vi "AlliGator Save Simulation Outputs to ASCII.vi"(8 "Error In":errorcluster, 11 "Fit Results":T1[](array[typedef])) -> (0 "Error Out":errorcluster)   [LabVIEW 2021, in "AlliGator Fit Method Benchmark.lvlib"]
doc: "Saves simulation results."
uses:
  AlliGator Fit Method Benchmark.lvlib
  Fits/IRF(X)PSED/IRF(X)PSED Fit Results.ctl
  Fits/IRF(X)PSED/Decay Fit Parameters & Derived Quantities List.ctl
  <vilib>/Utility/file.llb/Write Delimited Spreadsheet (DBL).vi
  Fits/Fits.lvlib
panel:
  out "Message":string
  # "see the AlliGator License on the block diagram (Ctrl+E or Window:Show Block Diagram)"
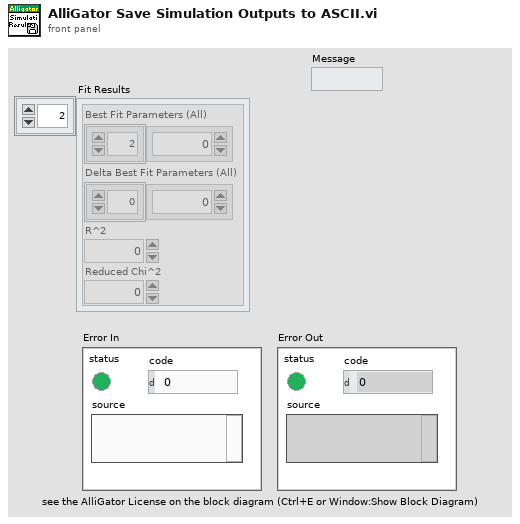
[diagram p1: front panel]
types:
  T1 = typedef "Fits.lvlib/IRF(X)PSED Fit Results.ctl" = cluster{"Best Fit Parameters (All)":dbl[], "Delta Best Fit Parameters (All)":dbl[], "R^2":dbl, "Reduced Chi^2":dbl}
  T2 = typedef "Fits.lvlib/Decay Fit Parameters & Derived Quantities List.ctl" = enum16{"Offset", "Baseline", "A_1", "tau_1", "A_2", "tau_2", "<tau>_a", "f1_a", "f2_a", "<tau>_i", "f1_i", "f2_i", "-", "R^2", "Chi^2"}
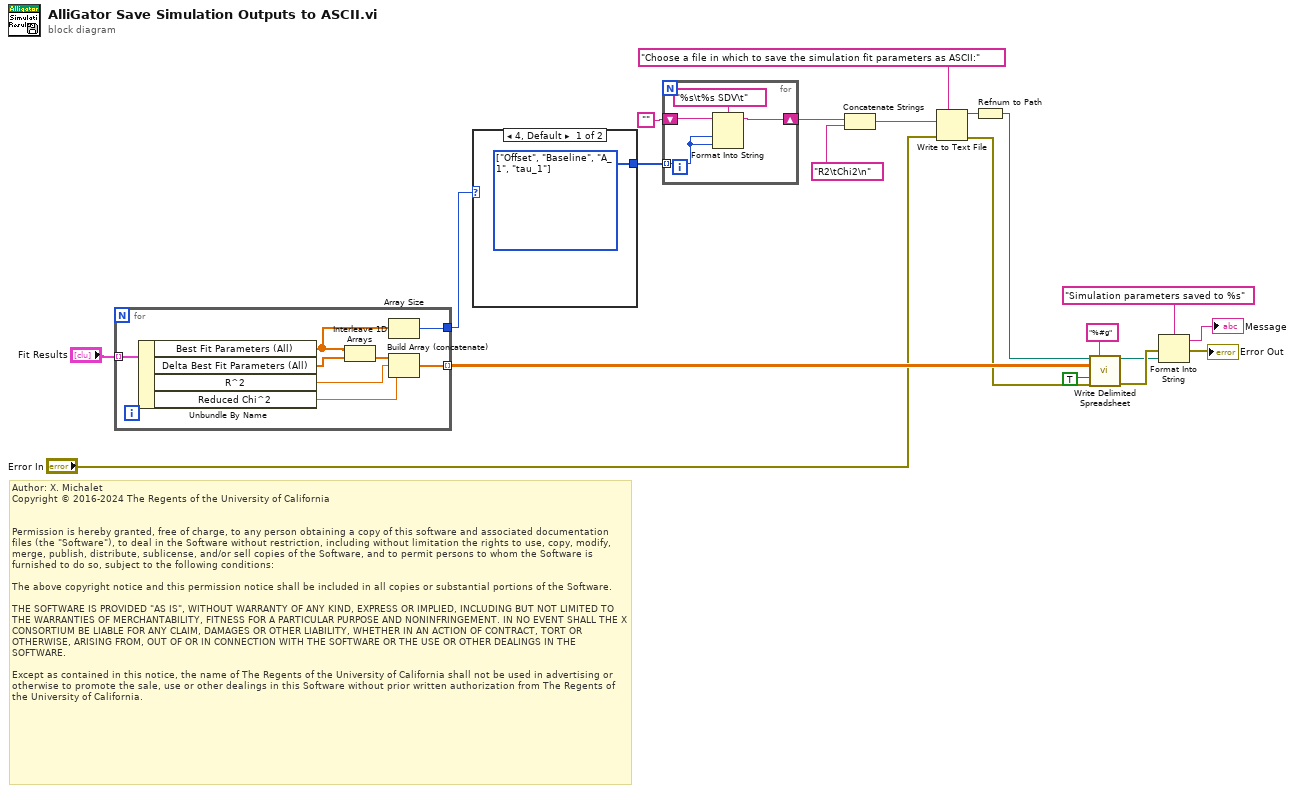
[diagram p0: block diagram]
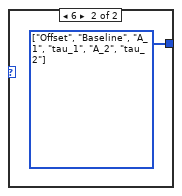
[diagram p2: hidden frame]
diagram:
  # "Author: X. Michalet\nCopyright © 2016-2024 The Regents of the University of California\n \n\nPermission is hereby granted, free of charge, to any person obtaining a copy of this software and associated documentation files (the \"Software\"), to deal in the Software without restriction, including without limitation the rights to use, copy, modify, merge, publish, distribute, sublicense, and/or sell copies of the Software, and to permit persons to whom the Software is furnished to do so, subject to the following conditions:\n\nThe above copyright notice and this permission notice shall be included in all copies or substantial portions of the Software.\n\nTHE SOFTWARE IS PROVIDED \"AS IS\", WITHOUT WARRANTY OF ANY KIND, EXPRESS OR IMPLIED, INCLUDING BUT NOT LIMITED TO THE WARRANTIES OF MERCHANTABILITY, FITNESS FOR A PARTICULAR PURPOSE AND NONINFRINGEMENT. IN NO EVENT SHALL THE X CONSORTIUM BE LIABLE FOR ANY CLAIM, DAMAGES OR OTHER LIABILITY, WHETHER IN AN ACTION OF CONTRACT, TORT OR OTHERWISE, ARISING FROM, OUT OF OR IN CONNECTION WITH THE SOFTWARE OR THE USE OR OTHER DEALINGS IN THE SOFTWARE.\n\nExcept as contained in this notice, the name of The Regents of the University of California shall not be used in advertising or otherwise to promote the sale, use or other dealings in this Software without prior written authorization from The Regents of the University of California."
  n1 = for {
    tunnel: "Fit Results" -> [w28] mode=indexing
    tunnel: [w23] -> w19 mode=indexing
    tunnel: [w21] -> w18
    n2 = Unbundle By Name(w28) -> ("Best Fit Parameters (All)"=w22:dbl[], "Delta Best Fit Parameters (All)"=w27:dbl[], "R^2"=w25:dbl, "Reduced Chi^2"=w24:dbl)
    n3 = Interleave 1D Arrays(w22, w27) -> (w26:dbl[])
    n4 = Array Size(array=w22) -> (size(s)=w21:i32)
    n5 = Build Array (concatenate)(w26, w25, w24) -> (w23:dbl[])
  }
  n6 = case shown="4, Default" w18 {
    tunnel: [w29 w30] -> w16
    frame 4, Default {
      w29 = T2[] [enum."Offset", enum."Baseline", enum."A_1", enum."tau_1"] items=["Offset", "Baseline", "A_1", "tau_1", "A_2", "tau_2", "<tau>_a", "f1_a", "f2_a", "<tau>_i", "f1_i", "f2_i", "-", "R^2", "Chi^2"] ("Array")
    }
    frame 6 {
      w30 = T2[] [enum."Offset", enum."Baseline", enum."A_1", enum."tau_1", enum."A_2", enum."tau_2"] items=["Offset", "Baseline", "A_1", "tau_1", "A_2", "tau_2", "<tau>_a", "f1_a", "f2_a", "<tau>_i", "f1_i", "f2_i", "-", "R^2", "Chi^2"] ("Array")
    }
  }
  n7 = for {
    shift-right: [w32] -> w15
    shift-left: "" -> [w34]
    tunnel: w16 -> [w31] mode=indexing
    n8 = Format Into String(format string="%s\t%s SDV\t", initial string=w34, w31, w31) -> (resulting string=w32:string)  [unwired: 1 in, 1 out]
  }
  n9 = Concatenate Strings(w15, "R2\tChi2\n" ("format string")) -> (w13:string)
  n10 = Write to Text File(prompt (Choose or enter file path)="Choose a file in which to save the simulation fit parameters as ASCII:", text=w13, error in="Error In") -> (refnum out=w10:refnum<file>, error out=w8:errorcluster)  [unwired: 1 in, 1 out]
  n11 = Refnum to Path(1:w10) -> (0:w9:path)
  n12 = call-poly <vilib>:"Write Delimited Spreadsheet.vi"("file path (dialog if empty)"=w9, "format (%.3f)"="%#g", "2D data"=w19, "append to file? (new file:F)"=TRUE ("transpose? (no:F)"), "error in (no error)"=w8) -> ("new file path (Not A Path if cancelled)"=w4:path, "error out"=w5:errorcluster)  [unwired: 9 in]
  n13 = Format Into String(format string="Simulation parameters saved to %s", error in=w5, w4) -> (resulting string=→"Message":string, error out=→"Error Out":errorcluster)  [unwired: 1 in]
